vi "Get Pin Command.vi"(7 "Marca":string, 8 "error in (no error)":errorcluster, 9 "Pin":string, 10 "Puerto":string, 11 "Serial Device in":refnum<class "Serial Device.lvclass">) -> (0 "error out":errorcluster, 1 "Expected response":string, 2 "Command":string, 3 "Serial Device out":refnum<class "Serial Device.lvclass">)   [LabVIEW 2020, in "Serial Device.lvclass"]
uses:
  Serial Device.lvclass
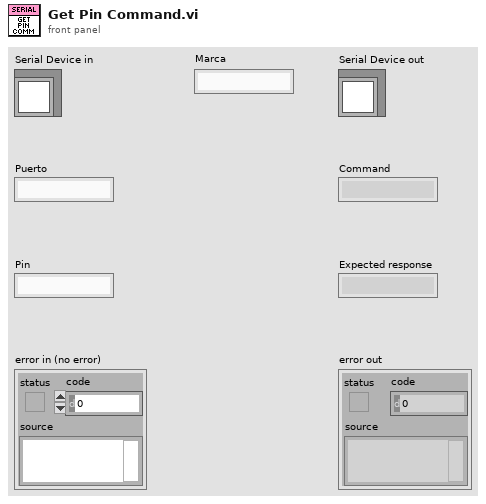
[diagram p1: front panel]
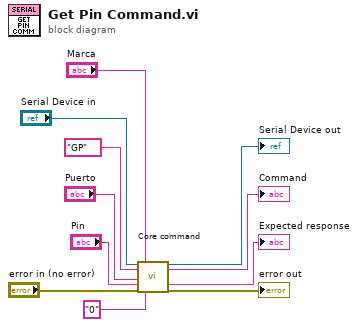
[diagram p0: block diagram]
diagram:
  n1 = call-dynamic "Core command.vi"("object in"="Serial Device in", "Command"="GP", "Param1"="Puerto", "Param2"="Pin", "error in (no error)"="error in (no error)", "Marca"="Marca", "Param3"="0") -> ("object out"=→"Serial Device out":refnum<class "Serial Device.lvclass">, "Command"=→"Command":string, "Expected response"=→"Expected response":string, "error out"=→"error out":errorcluster)  [unwired: 9 in]
